vi "Tektronix 7000 Series Histogram Measurement.vi"() -> ()   [LabVIEW 2015]
doc: "This example VI illustrates how to configure an oscilloscope to perform a measurement and create a corresponding histogram."
uses:
  <instrlib>/Tektronix 7000 Series/Public/Data/Read Waveform Measurement (Histogram).vi
  <instrlib>/Tektronix 7000 Series/Tektronix 7000 Series.lvlib
panel:
  in  "Maximum Time (25000ms)":u32=25000
  in  "Histogram Scaling (0:Linear)":u16(ring) items=["Linear", "Log"]
  out "Measurement":dbl
  in  "Channels (0:Channel1)":u16(ring) items=["Channel 1", "Channel 2", "Channel 3", "Channel 4", "Math 1", "Math 2", "Math 3", "Math 4", "Reference 1", "Reference 2", "Reference 3", "Reference 4"]
  in  "Histogram Type (0:Horizontal)":u16(ring) items=["Horizontal", "Vertical"]
  in  "Function (0:Wfm Ct)":u16(ring) items=["Wfm Ct", "Median", "Pk-Pk", "Hits in Box", "Max", "Mean", "Peak Hits", "Min", "St Dev", "Sigma1", "Sigma2", "Sigma3"]
  in  "Adjust Histogram Box":T1={"Left Limit (-0.001s)"=-0.001, "Top Limit (1.25V)"=1.25, "Right Limit (0.001s)"=0.001, "Bottom Limit (-1.25v)"=-1.25}
  in  "VISA Resource Name":refnum<visa-resource-name>
  # "(c) 2006 - 2016 National Instruments Corporation.  ALL RIGHTS RESERVED."
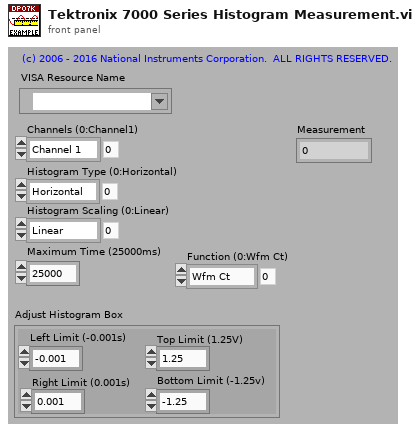
[diagram p1: front panel]
types:
  T1 = cluster{"Left Limit (-0.001s)":dbl, "Top Limit (1.25V)":dbl, "Right Limit (0.001s)":dbl, "Bottom Limit (-1.25v)":dbl}
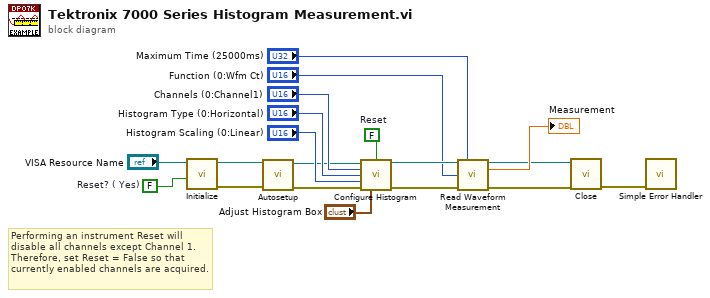
[diagram p0: block diagram]
diagram:
  w1 = FALSE  # Reset? ( Yes)
  w2 = FALSE  # Reset
  # "Performing an instrument Reset will disable all channels except Channel 1. Therefore, set Reset = False so that currently enabled channels are acquired."
  n1 = call <instrlib>:"Initialize.vi"("Reset? ( Yes)"=w1, "VISA resource name"="VISA Resource Name") -> ("error out"=w5:errorcluster, "VISA resource name out"=w6:refnum<visa-resource-name>)  [unwired: 8 in]
  n2 = call <instrlib>:"Autosetup.vi"("error in (no error)"=w5, "VISA resource name"=w6) -> ("error out"=w3:errorcluster, "VISA resource name out"=w4:refnum<visa-resource-name>)  [unwired: 8 in]
  n3 = call <instrlib>:"Configure Histogram.vi"("VISA resource name"=w4, "Reset (ON)"=w2, "Channels (0:Channel1)"="Channels (0:Channel1)", "Histogram Type (0:Horizontal)"="Histogram Type (0:Horizontal)", "Histogram Scaling (0:Linear)"="Histogram Scaling (0:Linear)", "error in (no error)"=w3, "Adjust Histogram Box"="Adjust Histogram Box") -> ("VISA resource name out"=w18:refnum<visa-resource-name>, "error out"=w17:errorcluster)  [unwired: 7 in]
  n4 = call-poly <instrlib>:"Read Waveform Measurement.vi"("VISA resource name"=w18, "Maximum Time (25000ms)"="Maximum Time (25000ms)", "Function (0:Wfm Ct)"="Function (0:Wfm Ct)", "error in (no error)"=w17) -> ("VISA resource name out"=w15:refnum<visa-resource-name>, "Measurement"=→"Measurement":dbl, "error out"=w14:errorcluster)  [unwired: 9 in]
  n5 = call <instrlib>:"Close.vi"("error in (no error)"=w14, "VISA resource name"=w15) -> ("error out"=w13:errorcluster)  [unwired: 9 in]
  n6 = call <vilib>:"Simple Error Handler.vi"("error in (no error)"=w13) -> ()  [unwired: 4 in, 5 out]
